vi "BRig_RT__Case_Exp__storeData__endExp__v5__p1.vi"(0 "input_dataCurrent":u16[](array[numeric]), 1 "input_dataLC":u16[](array[numeric]), 2 "input_dataExp":u16[](array[numeric]), 9 "input_dataExp_end":u16[](array[numeric]), 11 "input_dataLC_end":u16[](array[numeric])) -> (8 "output_True":bool)   [LabVIEW 2014]
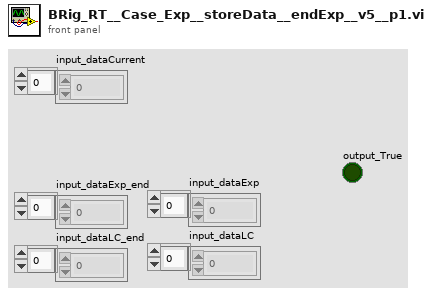
[diagram p1: front panel]
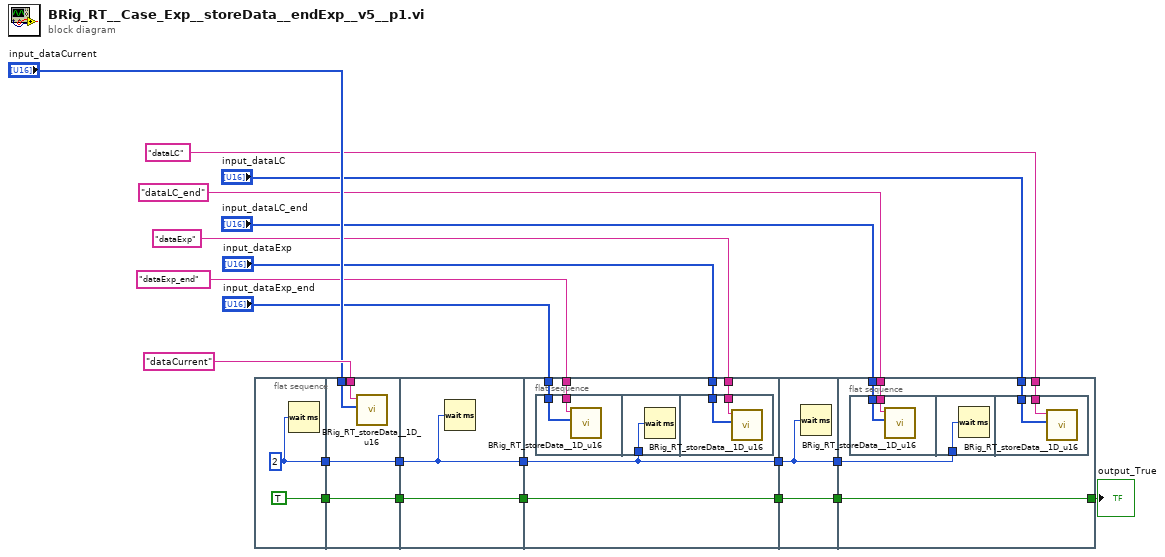
[diagram p0: block diagram]
diagram:
  n1 = flat-sequence {
    tunnel: [TRUE] -> w8
    tunnel: [w22] -> w7
    tunnel: "dataCurrent" ("input_filename") -> [w27]
    tunnel: "input_dataCurrent" -> [w26]
    tunnel: [w25] -> w10
    tunnel: w8 -> [w25]
    tunnel: w7 -> [w24]
    tunnel: [w24] -> w6
    tunnel: [w29] -> w11
    tunnel: w10 -> [w29]
    tunnel: w6 -> [w28]
    tunnel: [w28] -> w5
    tunnel: "input_dataExp_end" -> [w35]
    tunnel: "dataExp_end" ("input_filename") -> [w34]
    tunnel: "input_dataExp" -> [w33]
    tunnel: "dataExp" ("input_filename") -> [w32]
    tunnel: [w31] -> w4
    tunnel: w11 -> [w31]
    tunnel: w5 -> [w30]
    tunnel: [w30] -> w2
    tunnel: w4 -> [w42]
    tunnel: [w42] -> w3
    tunnel: w2 -> [w41]
    tunnel: [w41] -> w1
    tunnel: "input_dataLC_end" -> [w48]
    tunnel: "dataLC_end" ("input_filename") -> [w47]
    tunnel: "dataLC" ("input_filename") -> [w46]
    tunnel: "input_dataLC" -> [w45]
    tunnel: w3 -> [w44]
    tunnel: [w44] -> w9
    tunnel: w1 -> [w43]
    frame #0 {
      w22 = u32 2 ("milliseconds to wait")
      n2 = Wait (ms)(milliseconds to wait=w22) -> ()  [unwired: 1 out]
    }
    frame #1 {
      n3 = call "BRig_RT_storeData__1D_u16.vi"("Array"=w26, "input_filename"=w27) -> ()  [unwired: 10 in]
    }
    frame #2 {
      n4 = Wait (ms)(milliseconds to wait=w28) -> ()  [unwired: 1 out]
    }
    frame #3 {
      n5 = flat-sequence {
        tunnel: w35 -> [w37]
        tunnel: w34 -> [w36]
        tunnel: w30 -> [w38]
        tunnel: w33 -> [w39]
        tunnel: w32 -> [w40]
        frame #0 {
          n6 = call "BRig_RT_storeData__1D_u16.vi"("Array"=w37, "input_filename"=w36) -> ()  [unwired: 10 in]
        }
        frame #1 {
          n7 = Wait (ms)(milliseconds to wait=w38) -> ()  [unwired: 1 out]
        }
        frame #2 {
          n8 = call "BRig_RT_storeData__1D_u16.vi"("Array"=w39, "input_filename"=w40) -> ()  [unwired: 10 in]
        }
      }
    }
    frame #4 {
      n9 = Wait (ms)(milliseconds to wait=w41) -> ()  [unwired: 1 out]
    }
    frame #5 {
      n10 = flat-sequence {
        tunnel: w48 -> [w50]
        tunnel: w47 -> [w49]
        tunnel: w43 -> [w51]
        tunnel: w46 -> [w53]
        tunnel: w45 -> [w52]
        frame #0 {
          n11 = call "BRig_RT_storeData__1D_u16.vi"("Array"=w50, "input_filename"=w49) -> ()  [unwired: 10 in]
        }
        frame #1 {
          n12 = Wait (ms)(milliseconds to wait=w51) -> ()  [unwired: 1 out]
        }
        frame #2 {
          n13 = call "BRig_RT_storeData__1D_u16.vi"("Array"=w52, "input_filename"=w53) -> ()  [unwired: 10 in]
        }
      }
    }
  }
  "output_True" <- w9
